vi "TeleopServo.vi"(11 "Degrees":dbl) -> ()   [LabVIEW 2015]
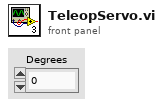
[diagram p1: front panel]
types:
  T1 = typedef "WPI_ServoDeviceRef.ctl" = cluster{"DeviceStatus":errorcluster, "PWM Channel":T2, "DeadBand":T3}
  T2 = typedef "FPGA_DIOPWMChannel.ctl" = enum8{"PWM 0", "PWM 1", "PWM 2", "PWM 3", "PWM 4", "PWM 5", "PWM 6", "PWM 7", "PWM 8", "PWM 9", "PWM MXP 0", "PWM MXP 1", "PWM MXP 2", "PWM MXP 3", "PWM MXP 4", "PWM MXP 5", "PWM MXP 6", "PWM MXP 7", "PWM MXP 8", "PWM MXP 9", "Invalid"}
  T3 = typedef "WPI_PWMDeadband.ctl" = cluster{"Name":string, "maxPositivePwm":i32, "minPositivePwm":i32, "centerPwm":i32, "maxNegativePwm":i32, "minNegativePwm":i32, "angularRange":u16}
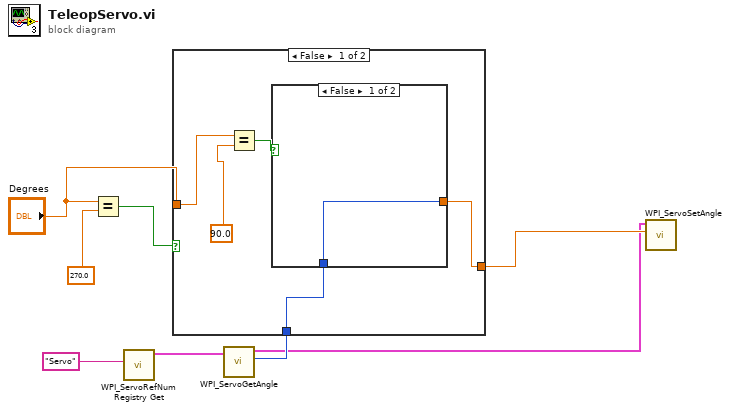
[diagram p0: block diagram]
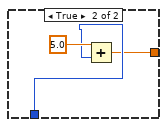
[diagram p2: hidden frame]
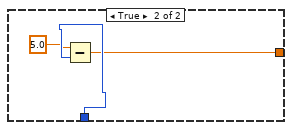
[diagram p3: hidden frame]
diagram:
  n1 = Equal?(x="Degrees", y=270.0) -> (x = y?=w4:bool)
  n2 = call <vilib>:"WPI_ServoRefNum Registry Get.vi"("refnum name"="Servo") -> ("ServoDeviceRef"=w7:T1)  [unwired: 9 in, 1 out]
  n3 = call <vilib>:"WPI_ServoGetAngle.vi"("ServoDeviceRef"=w7) -> ("ServoDeviceRef"=w1:T1, "Angle"=w6:u16)  [unwired: 7 in, 1 out]
  n4 = case shown="False" w4 {
    tunnel: w6 -> [w10 w20]
    tunnel: [w9 w18] -> w5
    tunnel: "Degrees" -> [w12 _]
    frame False {
      n5 = Equal?(x=w12, y=90.0) -> (x = y?=w11:bool)
      n6 = case shown="False" w11 {
        tunnel: w10 -> [w14 w16]
        tunnel: [w14 w15] -> w9
        frame False {
        }
        frame True {
          n7 = Add(x=5.0 ("y"), y=w16) -> (x+y=w15:dbl)
        }
      }
    }
    frame True {
      n8 = Subtract(x=5.0 ("y"), y=w20) -> (x-y=w18:dbl)
    }
  }
  n9 = call <vilib>:"WPI_ServoSetAngle.vi"("Angle"=w5, "ServoDeviceRef"=w1) -> ()  [unwired: 8 in, 2 out]
